vi "Upload Errors To File.vi"(6 "Station":string="St 65", 8 "error in":errorcluster, 9 "Error Table":string[][](array[string]), 10 "Serial Number":string, 11 "Path":path=path "C:/Labview Code") -> (0 "error out":errorcluster)   [LabVIEW 2018]
uses:
  02.Type Def's/Error Data Cluster 1.0.ctl
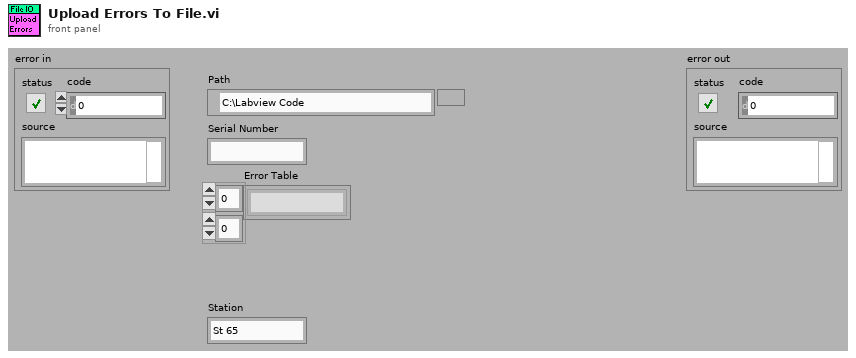
[diagram p1: front panel]
types:
  T1 = typedef "Error Data Cluster 1.0.ctl" = cluster{"Serial Number":string, "Error Data":string[], "Retry Counter":u8}
  T2 = cluster{"Error History":T1[], "Path":path, "Serial Number":string, "Index":i32}
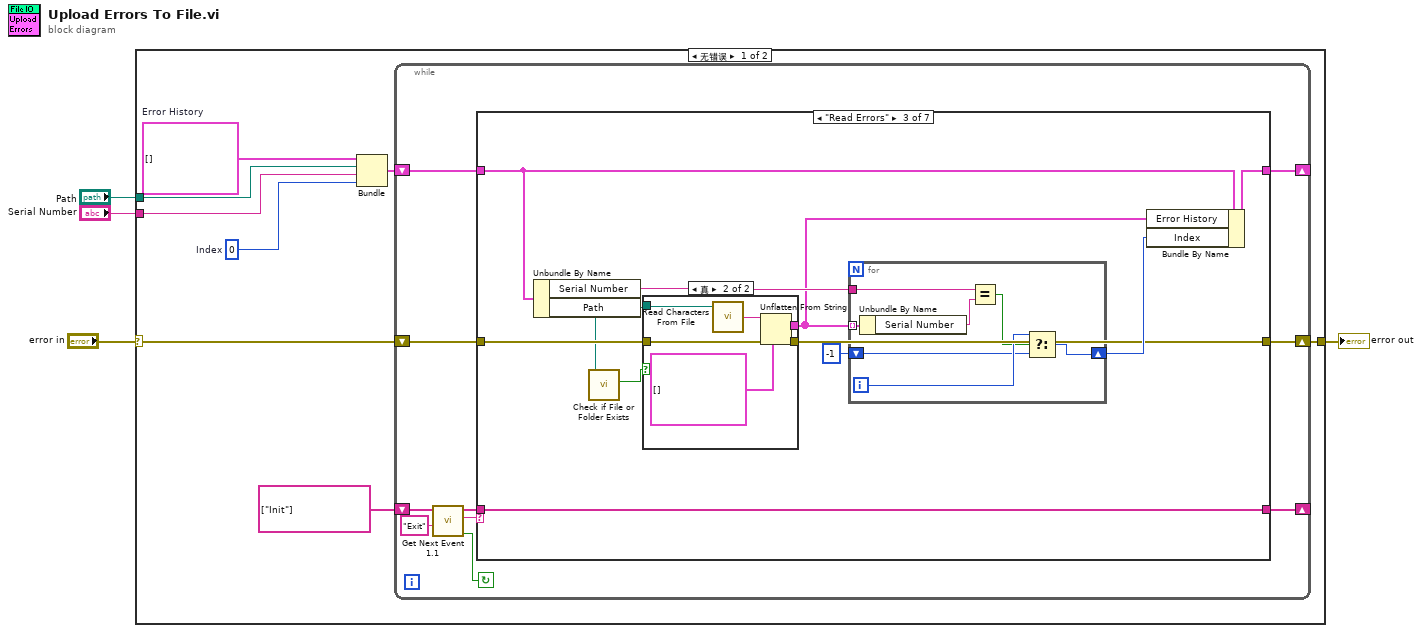
[diagram p0: block diagram]
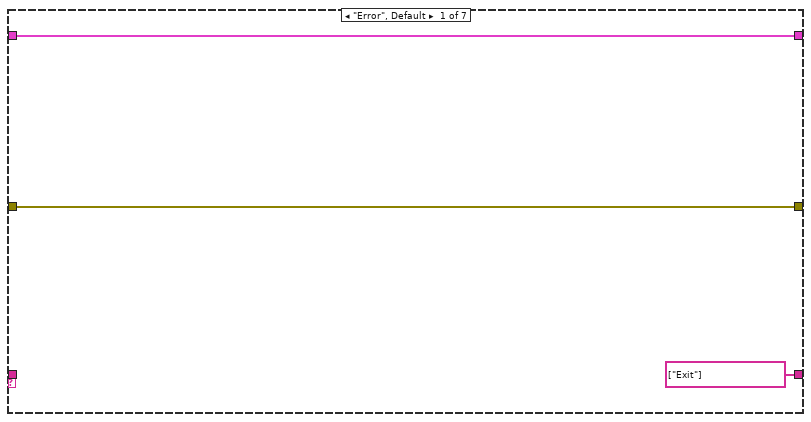
[diagram p2: hidden frame]
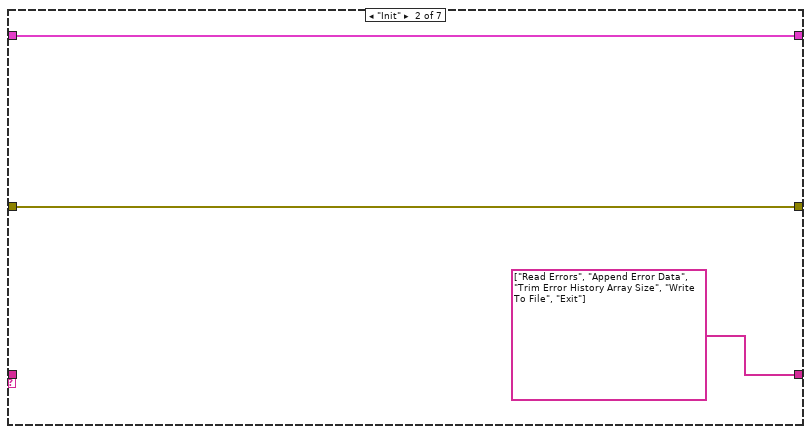
[diagram p3: hidden frame]
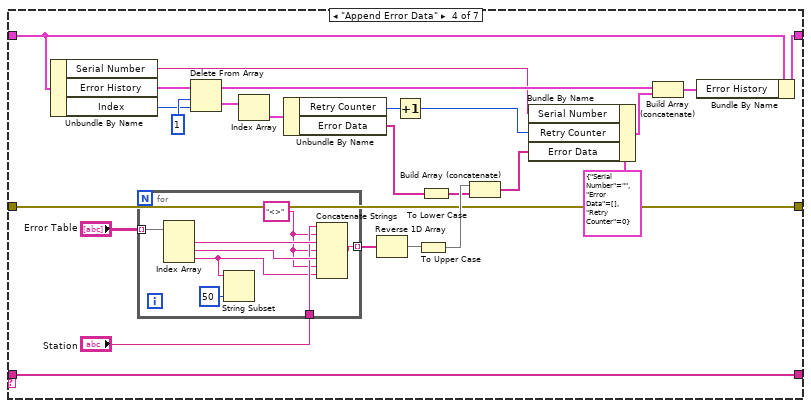
[diagram p5: hidden frame]
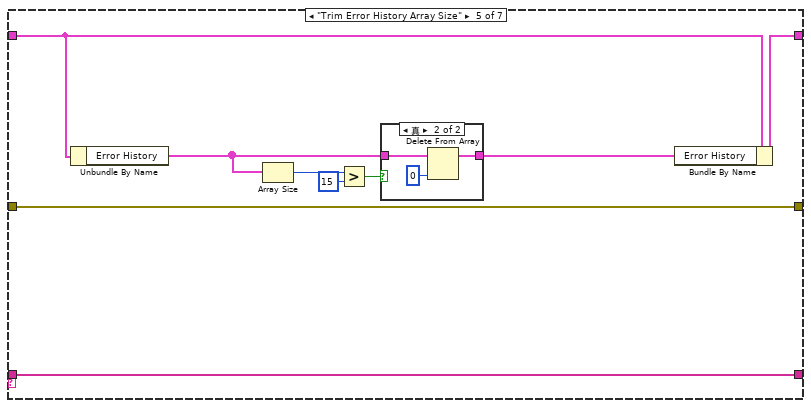
[diagram p6: hidden frame]
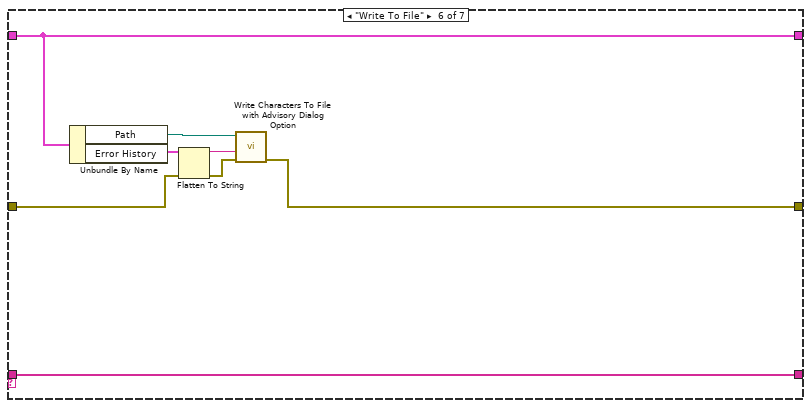
[diagram p8: hidden frame]
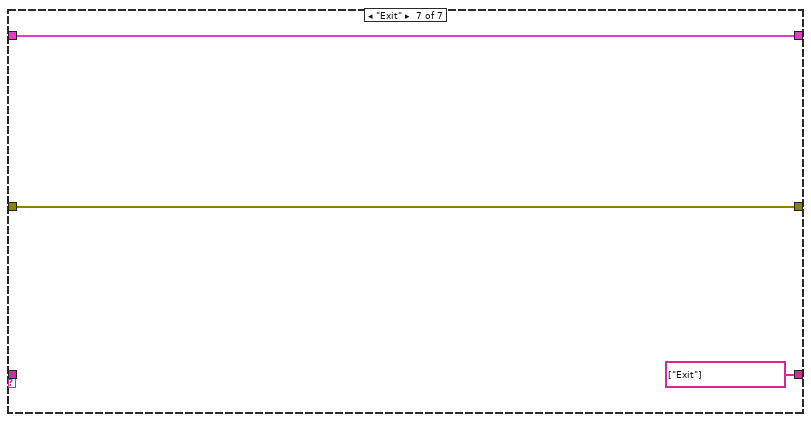
[diagram p9: hidden frame]
diagram:
  n1 = case shown="无错误" "error in" {
    selector: "error in" -> [w5 w110]
    tunnel: "Path" -> [w10 _]
    tunnel: "Serial Number" -> [w9 _]
    tunnel: [w6 w110] -> w2
    frame No Error {
      w7 = T1[] []  # Error History
      w8 = 0  # Index
      n2 = Bundle("Error History"=w7, "Path"=w10, "Serial Number"=w9, "Index"=w8) -> (w11:T2)  [unwired: 1 in]
      n3 = while {
        shift-right: [w19] -> _
        shift-left: string[] ["Init"] ("event queue out") -> [w18]
        shift-right: [w15] -> _
        shift-left: w11 -> [w16]
        shift-right: [w13] -> w6
        shift-left: w5 -> [w14]
        stop <- w22 continue-if-true
        n4 = call "Get Next Event 1.1.vi"("Exit Event"="Exit", "event queue in"=w18) -> ("Condition (Exit:F)"=w22:bool, "next event"=w21:string, "event queue out"=w20:string[])  [unwired: 6 in, 1 out]
        n5 = case shown="\"Read Errors\"" w21 {
          tunnel: w20 -> [_ _ w39 w77 w94 w106 _]
          tunnel: [string[] ["Exit"] ("event queue out") string[] ["Read Errors", "Append Error Data", "Trim Error History Array Size", "Write To File", "Exit"] ("event queue out") w39 w77 w94 w106 string[] ["Exit"] ("event queue out")] -> w19
          tunnel: w16 -> [w24 w27 w36 w58 w89 w105 w108]
          tunnel: [w24 w27 w35 w57 w88 w105 w108] -> w15
          tunnel: w14 -> [w23 w26 w32 w54 w86 w101 w107]
          tunnel: [w23 w26 w31 w54 w86 w99 w107] -> w13
          frame "Error", Default {
          }
          frame "Init" {
          }
          frame "Read Errors" {
            n6 = Unbundle By Name(w36) -> ("Serial Number"=w38:string, "Path"=w30:path)
            n7 = call <vilib>:"Check if File or Folder Exists.vi"("path"=w30) -> ("file or folder exists?"=w29:bool)  [unwired: 8 in, 2 out]
            n8 = case shown="真" w29 {
              tunnel: [_ w44] -> w33
              tunnel: w30 -> [_ w43]
              tunnel: w32 -> [w40 w42]
              tunnel: [w40 w41] -> w31
              frame False {
              }
              frame True {
                n9 = call <vilib>:"Read Characters From File.vi"("file path (dialog if empty)"=w43) -> ("character string"=w45:string)  [unwired: 5 in, 3 out]
                n10 = Unflatten From String(type=T1[] [], binary string=w45, error in (no error)=w42) -> (value=w44:T1[], error out=w41:errorcluster)  [unwired: 2 in, 1 out]
              }
            }
            n11 = for {
              tunnel: w33 -> [w53] mode=indexing
              tunnel: w38 -> [w51]
              shift-right: [w48] -> w34
              shift-left: -1 -> [w49]
              i -> [w50]
              n12 = Unbundle By Name(w53) -> ("Serial Number"=w52:string)
              n13 = Equal?(x=w51, y=w52) -> (x = y?=w47:bool)
              n14 = Select(t=w50, s=w47, f=w49) -> (s? t:f=w48:i32)
            }
            n15 = Bundle By Name(cluster=w36, "Error History"=w33, "Index"=w34) -> (w35:T2)
          }
          frame "Append Error Data" {
            n16 = Unbundle By Name(w58) -> ("Serial Number"=w62:string, "Error History"=w73:T1[], "Index"=w71:i32)
            n17 = for {
              tunnel: "Error Table" -> [w85] mode=indexing
              tunnel: [w82] -> w76 mode=indexing
              tunnel: "Station" -> [w80]
              w79 = "<>"
              n18 = Index Array(array=w85) -> (element #1=w84:string, element #2=w83:string, element #3=w78:string)  [unwired: 3 in]
              n19 = String Subset(string=w78, length (rest)=50 ("offset (0)")) -> ()  [unwired: 1 in, 1 out]
              n20 = Concatenate Strings(w80, w79, w84, w79, w83, w79, w78) -> (w82:string)
            }
            n21 = Delete From Array(array=w73, length=1, index=w71) -> (deleted portion=w70:T1[], array with subset deleted=w63:T1[])
            n22 = Index Array(array=w70) -> (element=w69:T1)  [unwired: 1 in]
            n23 = Unbundle By Name(w69) -> ("Retry Counter"=w67:u8, "Error Data"=w68:string[])
            n24 = Reverse 1D Array(array=w76) -> (reversed array=w66:string[])
            n25 = Increment(x=w67) -> (x+1=w61:u8)
            n26 = To Upper Case(1:w66) -> (0:w65:string[])
            n27 = To Lower Case(string=w68) -> (all lower case string=w64:string[])
            n28 = Build Array (concatenate)(w65, w64) -> (w55:string[])
            n29 = Bundle By Name(cluster=T1 {"Serial Number"="", "Error Data"=[], "Retry Counter"=0} ("element"), "Serial Number"=w62, "Retry Counter"=w61, "Error Data"=w55) -> (w59:T1)
            n30 = Build Array (concatenate)(w63, w59) -> (w56:T1[])
            n31 = Bundle By Name(cluster=w58, "Error History"=w56) -> (w57:T2)
          }
          frame "Trim Error History Array Size" {
            n32 = Unbundle By Name(w89) -> ("Error History"=w90:T1[])
            n33 = Array Size(array=w90) -> (size(s)=w93:i32)
            n34 = Greater?(x=w93, y=15) -> (0:w91:bool)
            n35 = case shown="真" w91 {
              tunnel: w90 -> [w95 w98]
              tunnel: [w95 w97] -> w87
              frame False {
              }
              frame True {
                n36 = Delete From Array(array=w98, index=0) -> (array with subset deleted=w97:T1[])  [unwired: 1 in, 1 out]
              }
            }
            n37 = Bundle By Name(cluster=w89, "Error History"=w87) -> (w88:T2)
          }
          frame "Write To File" {
            n38 = Unbundle By Name(w105) -> ("Path"=w102:path, "Error History"=w103:T1[])
            n39 = Flatten To String(anything=w103, error in (no error)=w101) -> (data string=w104:string, error out=w100:errorcluster)  [unwired: 2 in, 1 out]
            n40 = call "Write Characters To File with Advisory Dialog Option.vi"("error in"=w100, "character string"=w104, "file path (dialog if empty)"=w102) -> ("error out"=w99:errorcluster)  [unwired: 7 in, 1 out]
          }
          frame "Exit" {
          }
        }
      }
    }
    frame Error {
    }
  }
  "error out" <- w2
